vi "worksheet insert textbox opt lv.vi"(6 "options":T1, 7 "text":string, 8 "error in (no error)":errorcluster, 9 "col":u16, 10 "row":u32, 11 "worksheet":u32) -> (0 "error out":errorcluster, 3 "function return":u32(ring), 4 "options out":T1)   [LabVIEW 8.6]
doc: "lxw_error worksheet_insert_textbox_opt_lv(lxw_worksheet worksheet, lxw_row_t row, lxw_col_t col, const char *text, lxw_textbox_options *options);"
uses:
  pending_lvxlsxwriter/xlsxwriter.dll
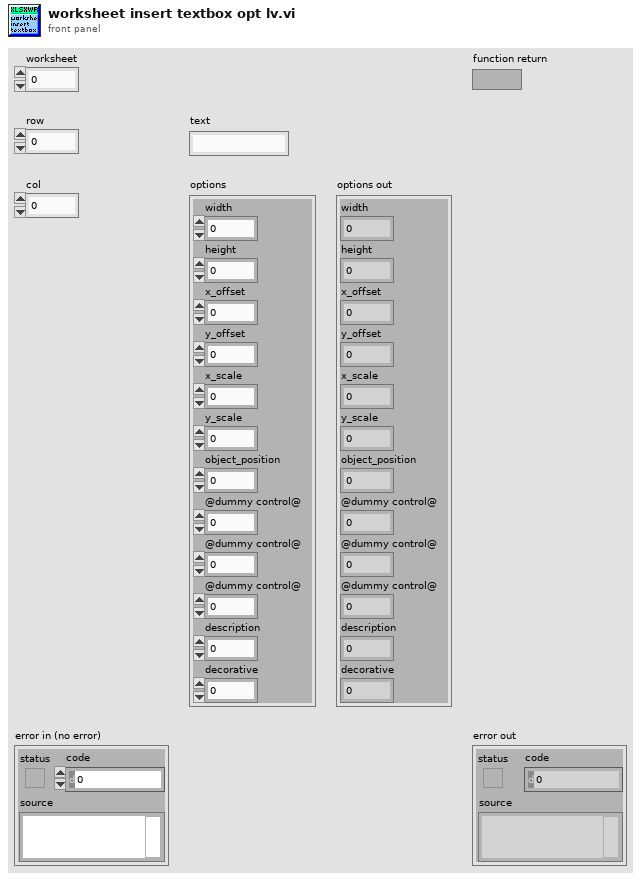
[diagram p1: front panel]
types:
  T1 = cluster{"width":u32, "height":u32, "x_offset":i32, "y_offset":i32, "x_scale":dbl, "y_scale":dbl, "object_position":u8, "@dummy control@":i8, "@dummy control@":i8, "@dummy control@":i8, "description":u32, "decorative":u8}
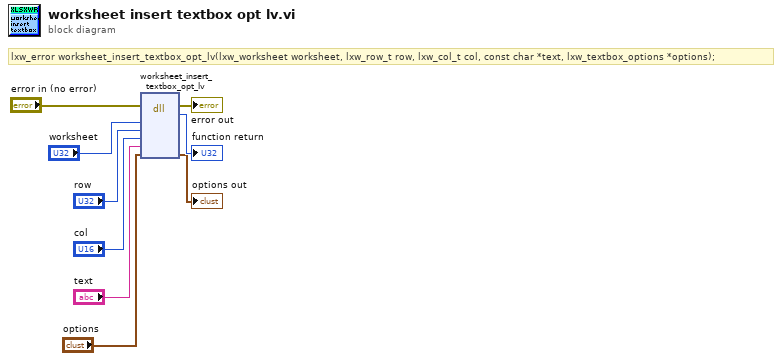
[diagram p0: block diagram]
diagram:
  # "lxw_error worksheet_insert_textbox_opt_lv(lxw_worksheet worksheet, lxw_row_t row, lxw_col_t col, const char *text, lxw_textbox_options *options);"
  n1 = dll-call lib="C:/Users/WDAGUtilityAccount/Desktop/pending_lvxlsxwriter/xlsxwriter.*" fn="worksheet_insert_textbox_opt_lv"(error in="error in (no error)", "worksheet"="worksheet", "row"="row", "col"="col", "text"="text", "options"="options") -> (error out=→"error out":errorcluster, →"function return":u32, "options"=→"options out":T1)  [unwired: 6 in, 1 out]
